vi "NI-XNET Frame&Log - Convert CAN to RAW.vi"(9 "CAN frame":T1 {"payload" format="%x"; "timestamp" format="%<%.7X\n%x>T"; "type" items=["CAN Data"=0, "CAN Remote"=1, "CAN Bus Error"=2, "Delay"=224, "Log Trigger"=225, "Start Trigger"=226]; "identifier" format="%x"}, 11 "error in":errorcluster) -> (8 "Raw Frame":u8[](array[numeric]), 15 "error out":errorcluster)   [LabVIEW 2014]
doc: "Convert a single CAN frame to insert into array of raw frame data."
uses:
  <vilib>/xnet/xnet.llb/XNET Frame CAN.ctl
  <vilib>/xnet/xnet.llb/XNET Frame Type CAN.ctl
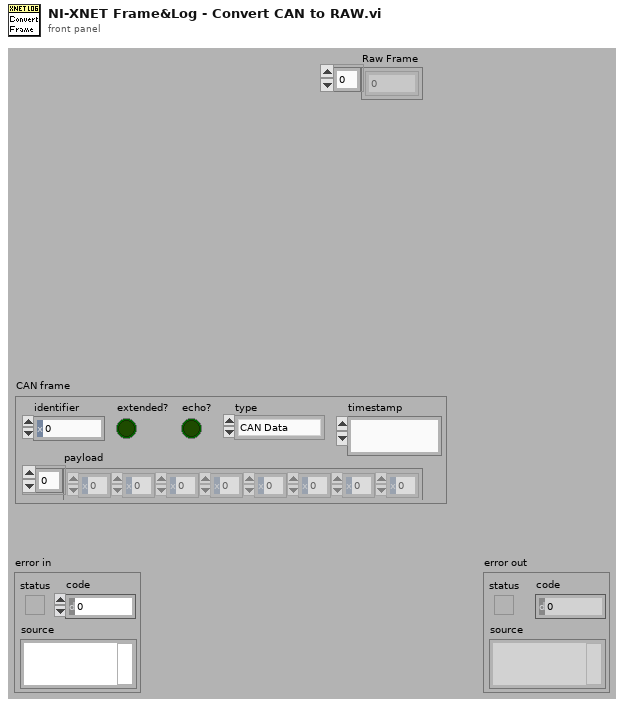
[diagram p1: front panel]
types:
  T1 = typedef "XNET Frame CAN.ctl" = cluster{"timestamp":timestamp, "payload":u8[], "identifier":u32, "type":T2, "extended?":bool, "echo?":bool}
  T2 = typedef "XNET Frame Type CAN.ctl" = u8
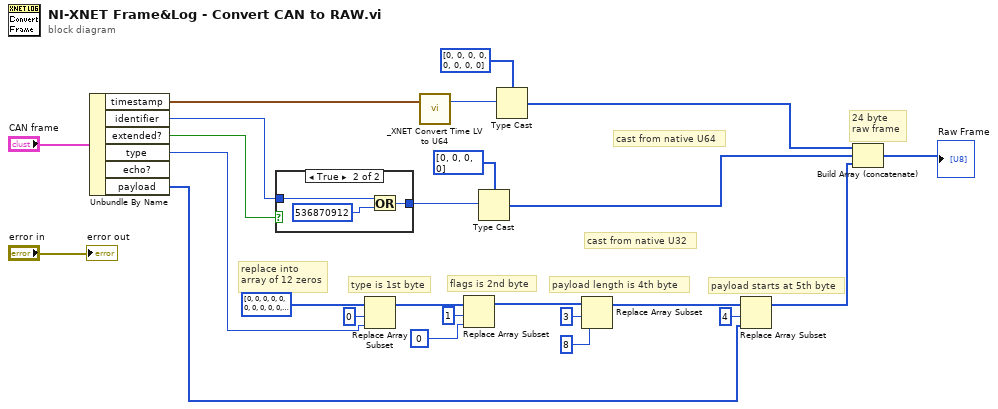
[diagram p0: block diagram]
diagram:
  # "flags is 2nd byte"
  # "24 byte\nraw frame"
  # "payload starts at 5th byte"
  # "payload length is 4th byte"
  # "type is 1st byte"
  # "replace into\narray of 12 zeros"
  # "cast from native U32"
  # "cast from native U64"
  n1 = Unbundle By Name("CAN frame") -> ("timestamp"=w21:timestamp, "identifier"=w23:u32, "extended?"=w22:bool, "type"=w18:T2, "payload"=w10:u8[])  [unwired: 1 out]
  n2 = case shown="True" w22 {
    tunnel: w23 -> [w26 w28]
    tunnel: [w26 w27] -> w1
    frame False {
    }
    frame True {
      n3 = Or(x=w28, y=u32 536870912) -> (x .or. y?=w27:u32)
    }
  }
  n4 = Replace Array Subset(array=u8[] [0, 0, 0, 0, 0, 0, 0, 0, 0, 0, 0, 0], new element=w18, index=0) -> (w12:u8[])
  n5 = call <vilib>:"_XNET Convert Time LV to U64.vi"("Time LV"=w21) -> ("Time U64"=w6:u64)  [unwired: 2 out]
  n6 = Replace Array Subset(array=w12, new element=u8 0 ("index"), index=1) -> (w11:u8[])
  n7 = Type Cast(type=u8[] [0, 0, 0, 0], x=w1) -> (*(type *) &x=w7:u8[])
  n8 = Type Cast(type=u8[] [0, 0, 0, 0, 0, 0, 0, 0], x=w6) -> (*(type *) &x=w4:u8[])
  n9 = Replace Array Subset(array=w11, new element=u8 8 ("new element/subarray"), index=3) -> (w15:u8[])
  n10 = Replace Array Subset(array=w15, new element=w10, index=4) -> (w14:u8[])
  n11 = Build Array (concatenate)(w4, w7, w14) -> (→"Raw Frame":u8[])
  "error out" <- "error in"
